vi "Update AI (SubVI).vi"(7 "Save":T1, 8 "error in (no error)":errorcluster, 9 "Value":dbl, 10 "AI_tasks":refnum<k21>, 11 "DaqPad_NI6009 in":refnum<class "DaqPad_NI6009.lvclass">) -> (0 "error out":errorcluster, 2 "String":string, 3 "DaqPad_NI6009 out":refnum<class "DaqPad_NI6009.lvclass">)   [LabVIEW 2020, in "DaqPad_NI6009.lvclass"]
uses:
  DaqPad_NI6009.lvclass
  OnOffTypeDef.ctl
  DaqPad_NI6009.lvclass/DaqPad_NI6009.ctl
  <resource>/objmgr/daqmx.rc
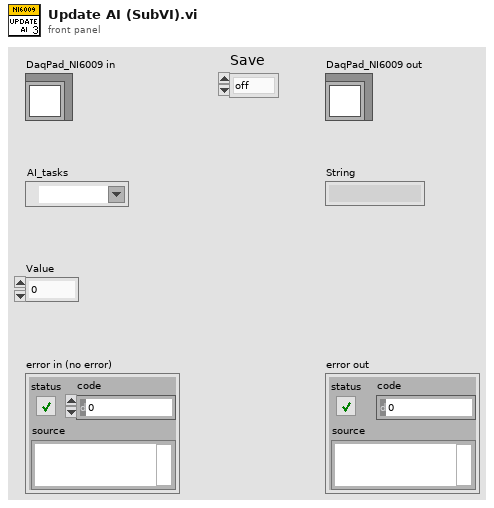
[diagram p1: front panel]
types:
  T1 = typedef "OnOffTypeDef.ctl" = enum16{"off", "on"}
  T2 = cluster{"Channel 0":dbl[], "Channel 1":dbl[], "Channel 2":dbl[], "Channel 3":dbl[], "Channel 4":dbl[], "Channel 5":dbl[], "Channel 6":dbl[], "Channel 7":dbl[], "Channel 8":dbl[], "Channel 9":dbl[], "Channel 10":dbl[], "Channel 11":dbl[], "Channel 12":dbl[], "Channel 13":dbl[], "Channel 14":dbl[], "Channel 15":dbl[], "Channel 16":dbl[], "Channel 17":dbl[], "Channel 18":dbl[], "Channel 19":dbl[], "Channel 20":dbl[], "Channel 21":dbl[], "Channel 22":dbl[], "Channel 23":dbl[], "Channel 24":dbl[], "Channel 25":dbl[], "Channel 26":dbl[], "Channel 27":dbl[], "Channel 28":dbl[], "Channel 29":dbl[], "Channel 30":dbl[], "Channel 31":dbl[]}
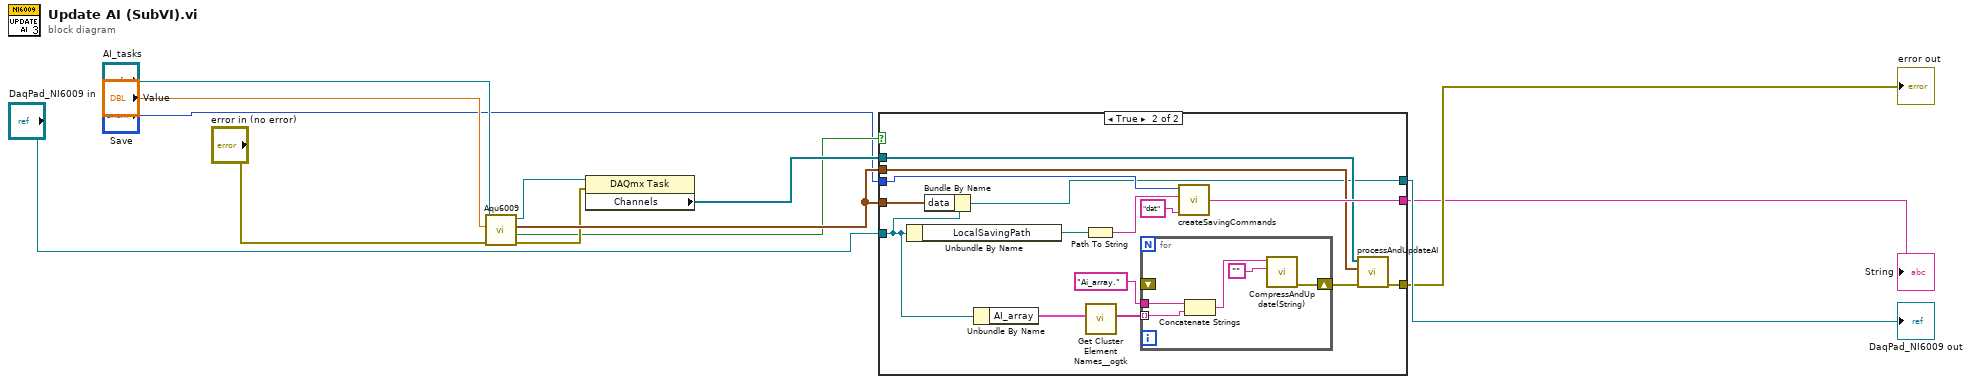
[diagram p0: block diagram]
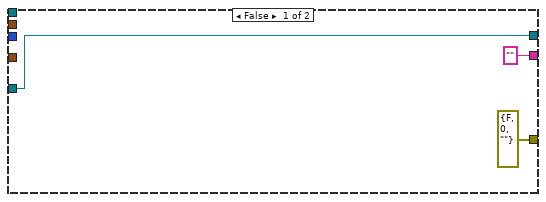
[diagram p2: hidden frame]
diagram:
  n1 = call "Aqu6009.vi"("error in (no error)"="error in (no error)", "timeout"="Value", "Refnum in"="AI_tasks") -> ("error out"=w9:errorcluster, "OK"=w6:bool, "data 2"=w10:waveform(dbl)[], "Refnum out"=w7:refnum<k21>)  [unwired: 5 in]
  n2 = property class="DAQmx Task"(reference=w7, error in=w9) -> ("Channels"=w8:refnum<k21>[])  [unwired: 2 out]
  n3 = case shown="True" w6 {
    tunnel: "Save" -> [_ w31]
    tunnel: "DaqPad_NI6009 in" -> [w14 w21]
    tunnel: ["" ("String") w27] -> w2
    tunnel: [errorcluster {"status"=FALSE, "code"=0, "source"=""} ("error IO") w25] -> w3
    tunnel: [w14 w22] -> w4
    tunnel: w10 -> [_ w24]
    tunnel: w8 -> [_ w26]
    tunnel: w10 -> [_ w23]
    frame False {
    }
    frame True {
      n4 = Unbundle By Name(w21) -> ("LocalSavingPath"=w28:path)
      n5 = Bundle By Name(cluster=w21, "data"=w23) -> (w22:refnum<class "DaqPad_NI6009.lvclass">)
      n6 = Unbundle By Name(w21) -> ("AI_array"=w20:T2)
      n7 = Path To String(path=w28) -> (string=w29:string)
      n8 = call "Get Cluster Element Names__ogtk.vi"("Cluster"=w20) -> ("Element Names"=w19:string[])  [unwired: 9 in, 1 out]
      n9 = for {
        tunnel: w19 -> [w36] mode=indexing
        tunnel: "Ai_array." ("string") -> [w35]
        shift-right: [w32] -> w17
        shift-left: _ -> [_]
        n10 = Concatenate Strings(w35, w36) -> (w34:string)
        n11 = call "CompressAndUpdate(String).vi"("String"="", "command or variable name"=w34) -> ("error out"=w32:errorcluster)  [unwired: 9 in]
      }
      n12 = call "createSavingCommands.vi"("extension"="dat" ("Fileextension"), "Saving Path (local)"=w29, "Save"=w31) -> ("String"=w27:string)  [unwired: 1 in]
      n13 = call "processAndUpdateAI.vi"("error in (no error)"=w17, "data in"=w24, "Channels"=w26) -> ("error out"=w25:errorcluster)  [unwired: 8 in]
    }
  }
  "DaqPad_NI6009 out" <- w4
  "error out" <- w3
  "String" <- w2
